vi "File.Read From CSV.vi"(8 "error in":errorcluster, 11 "File":path) -> (0 "error out":errorcluster, 2 "Data":string[][](array[string]), 3 "Header":string[](array[string]))   [LabVIEW 2024, in "EQMF.lvlib" / "File Utils.lvlib"]
uses:
  File Utils.lvlib
  <vilib>/Utility/error.llb/Trim Whitespace One-Sided.vi
panel:
  in  "Has Header Row":bool=TRUE
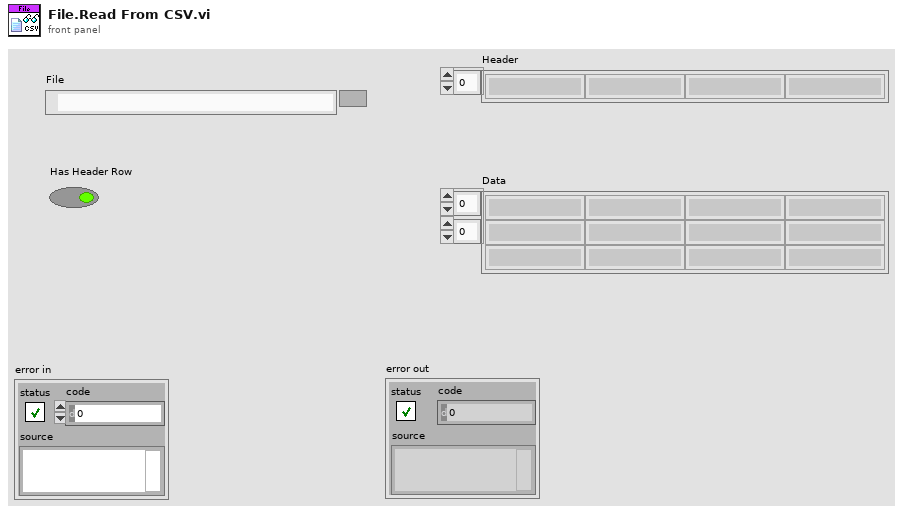
[diagram p1: front panel]
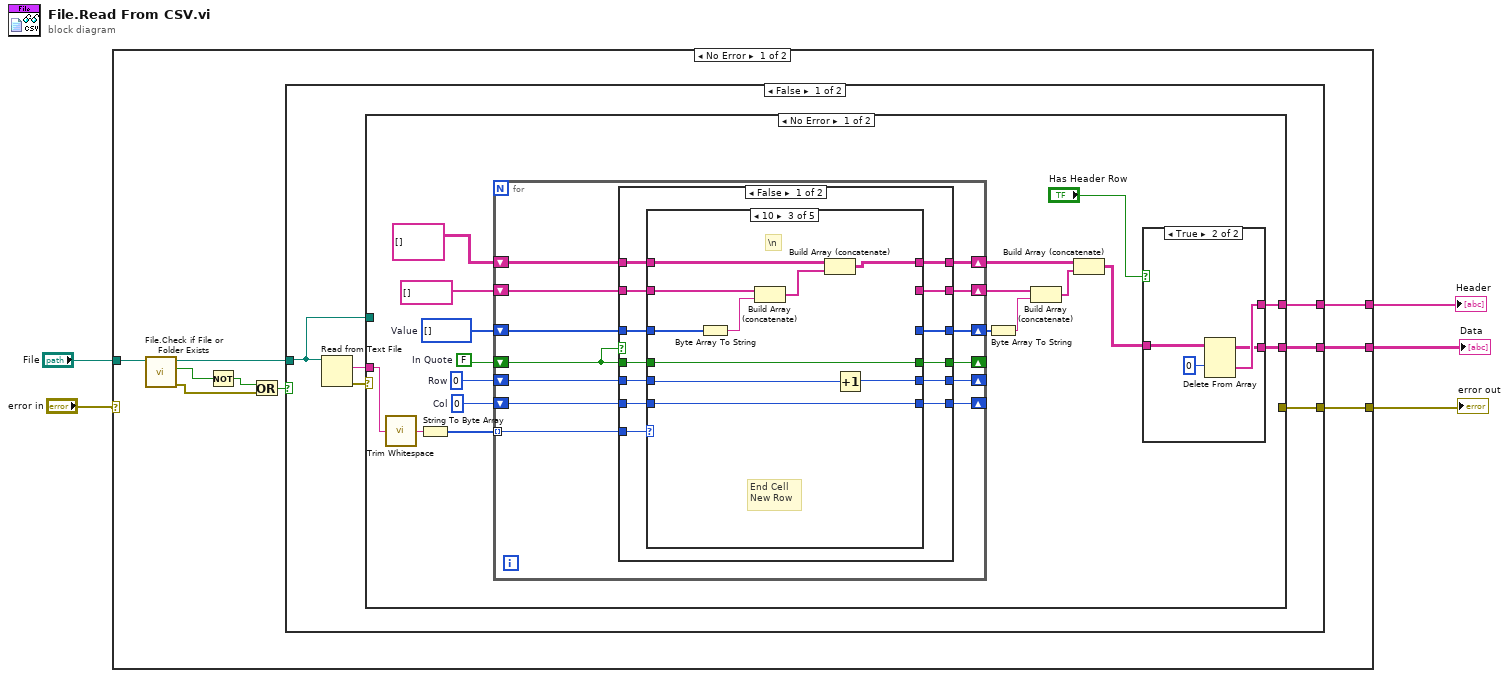
[diagram p0: block diagram]
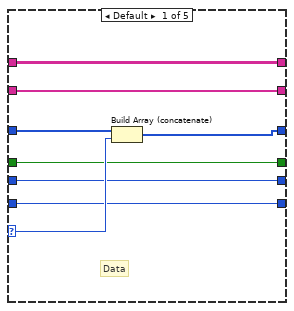
[diagram p2: hidden frame]
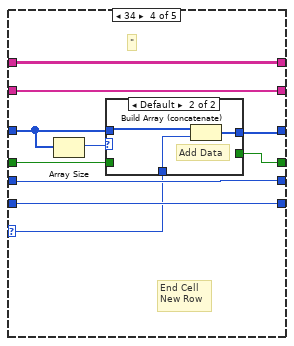
[diagram p4: hidden frame]
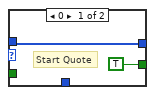
[diagram p5: hidden frame]
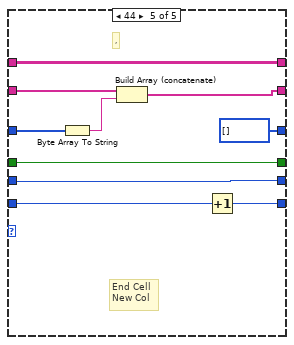
[diagram p6: hidden frame]
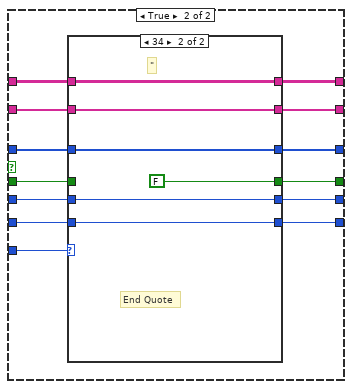
[diagram p7: hidden frame]
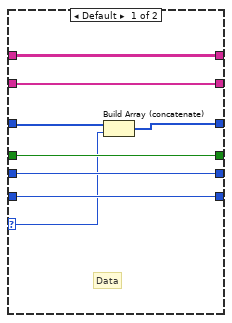
[diagram p8: hidden frame]
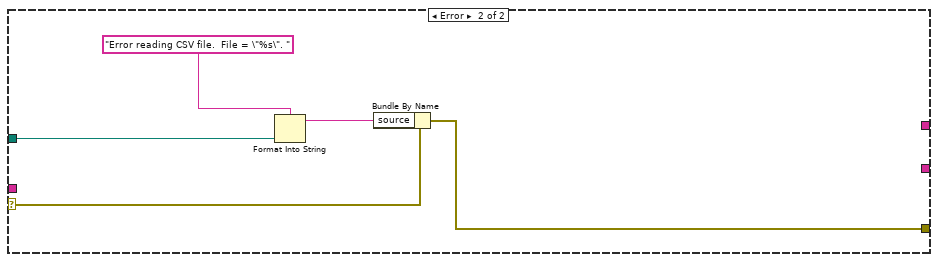
[diagram p10: hidden frame]
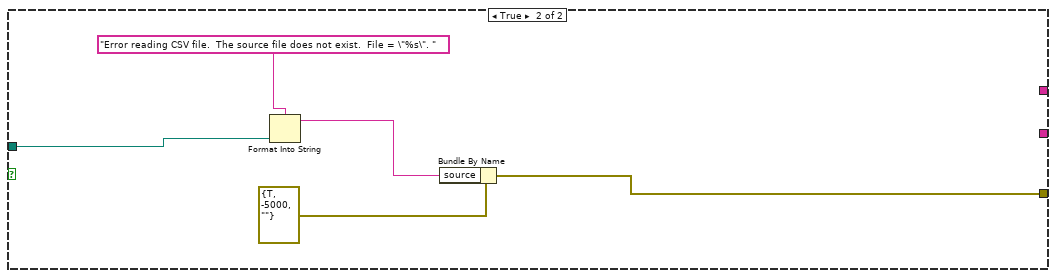
[diagram p11: hidden frame]
diagram:
  n1 = case shown="No Error" "error in" {
    selector: "error in" -> [_ w156]
    tunnel: "File" -> [w14 _]
    tunnel: [w8 w156] -> w3
    tunnel: [w7 _] -> w2
    tunnel: [w6 _] -> w1
    frame No Error {
      n2 = call "File.Check if File or Folder Exists.vi"("Path"=w14) -> ("error out"=w13:errorcluster, "Exists"=w10:bool, "Dup Path"=w11:path)  [unwired: 6 in, 2 out]
      n3 = Not(x=w10) -> (.not. x?=w12:bool)
      n4 = Or(x=w12, y=w13) -> (x .or. y?=w9:bool)
      n5 = case shown="False" w9 {
        tunnel: w11 -> [w18 w154]
        tunnel: [w17 w151] -> w8
        tunnel: [w16 _] -> w7
        tunnel: [w15 _] -> w6
        frame False {
          n6 = Read from Text File(file (use dialog)=w18) -> (text=w19:string, error out=w20:errorcluster)  [unwired: 3 in, 2 out]
          n7 = case shown="No Error" w20 {
            selector: w20 -> [_ w147]
            tunnel: w19 -> [w25 _]
            tunnel: w18 -> [_ w149]
            tunnel: [_ w146] -> w17
            tunnel: [w37 _] -> w16
            tunnel: [w36 _] -> w15
            frame No Error {
              w31 = FALSE  # In Quote
              w32 = u8[] []  # Value
              w33 = 0  # Col
              w34 = 0  # Row
              n8 = call <vilib>:"Trim Whitespace.vi"("string"=w25) -> ("trimmed string"=w26:string)  [unwired: 1 in]
              n9 = String To Byte Array(string=w26) -> (unsigned byte array=w27:u8[])
              n10 = for {
                tunnel: w27 -> [w44] mode=indexing
                shift-right: [w46] -> _
                shift-left: w33 -> [w50]
                shift-right: [w47] -> _
                shift-left: w34 -> [w51]
                shift-right: [w48] -> w23
                shift-left: w32 -> [w49]
                shift-right: [w45] -> _
                shift-left: w31 -> [w43]
                shift-right: [w41] -> w29
                shift-left: string[][] [] ("Raw") -> [w42]
                shift-right: [w40] -> w22
                shift-left: string[] [] ("Raw") -> [w39]
                n11 = case shown="False" w43 {
                  tunnel: w51 -> [w61 w124]
                  tunnel: w50 -> [w60 w122]
                  tunnel: w49 -> [w62 w126]
                  tunnel: [w57 w125] -> w48
                  tunnel: [w56 w123] -> w47
                  tunnel: [w53 w121] -> w46
                  tunnel: [w54 w120] -> w45
                  tunnel: w44 -> [w52 w114]
                  tunnel: w43 -> [w55 w119]
                  tunnel: w42 -> [w64 w116]
                  tunnel: [w63 w115] -> w41
                  tunnel: w39 -> [w58 w118]
                  tunnel: [w59 w117] -> w40
                  frame False {
                    n12 = case shown="10" w52 {
                      selector: w52 -> [w68 _ _ w90 _]
                      tunnel: w64 -> [w72 w78 w88 w96 w109]
                      tunnel: [w72 w78 w87 w96 w109] -> w63
                      tunnel: w62 -> [w70 w73 w79 w94 w110]
                      tunnel: w61 -> [w67 w76 w84 w97 w107]
                      tunnel: w60 -> [w66 w75 w83 w98 w105]
                      tunnel: w58 -> [w71 w77 w81 w95 w111]
                      tunnel: [w71 w77 _ w95 w108] -> w59
                      tunnel: [w69 w73 _ w91 u8[] [] ("Value")] -> w57
                      tunnel: [w67 w76 w85 w97 w107] -> w56
                      tunnel: w55 -> [w65 w74 w86 w92 w113]
                      tunnel: [w65 w74 w86 w89 w113] -> w54
                      tunnel: [w66 w75 w83 w98 w106] -> w53
                      frame Default {
                        # "Data"
                        n13 = Build Array (concatenate)(w70, w68) -> (w69:u8[])
                      }
                      frame 0..9, 11..31 {
                        # "Ignore"
                      }
                      frame 10 {
                        # "\\n"
                        # "End Cell\nNew Row"
                        n14 = Byte Array To String(unsigned byte array=w79) -> (string=w82:string)
                        n15 = Build Array (concatenate)(w81, w82) -> (w80:string[])
                        n16 = Build Array (concatenate)(w88, w80) -> (w87:string[][])
                        n17 = Increment(x=w84) -> (x+1=w85:i32)
                      }
                      frame 34 {
                        # "\""
                        # "End Cell\nNew Row"
                        n18 = Array Size(array=w94) -> (size(s)=w93:i32)
                        n19 = case shown="Default" w93 {
                          tunnel: w94 -> [w99 w103]
                          tunnel: w92 -> [_ _]
                          tunnel: [w99 w102] -> w91
                          tunnel: w90 -> [_ w101]
                          tunnel: [TRUE _] -> w89
                          frame 0 {
                            # "Start Quote"
                          }
                          frame Default {
                            # "Add Data"
                            n20 = Build Array (concatenate)(w103, w101) -> (w102:u8[])
                          }
                        }
                      }
                      frame 44 {
                        # ","
                        # "End Cell\nNew Col"
                        n21 = Byte Array To String(unsigned byte array=w110) -> (string=w112:string)
                        n22 = Build Array (concatenate)(w111, w112) -> (w108:string[])
                        n23 = Increment(x=w105) -> (x+1=w106:i32)
                      }
                    }
                  }
                  frame True {
                    n24 = case shown="34" w114 {
                      selector: w114 -> [w127 _]
                      tunnel: w126 -> [w132 w140]
                      tunnel: [w131 w140] -> w125
                      tunnel: w124 -> [w133 w139]
                      tunnel: [w133 w139] -> w123
                      tunnel: w122 -> [w134 w138]
                      tunnel: [w134 w138] -> w121
                      tunnel: [w130 FALSE] -> w120
                      tunnel: w119 -> [w130 _]
                      tunnel: w118 -> [w128 w136]
                      tunnel: [w128 w136] -> w117
                      tunnel: w116 -> [w129 w135]
                      tunnel: [w129 w135] -> w115
                      frame Default {
                        # "Data"
                        n25 = Build Array (concatenate)(w132, w127) -> (w131:u8[])
                      }
                      frame 34 {
                        # "\""
                        # "End Quote"
                      }
                    }
                  }
                }
              }
              n26 = Byte Array To String(unsigned byte array=w23) -> (string=w24:string)
              n27 = Build Array (concatenate)(w22, w24) -> (w21:string[])
              n28 = Build Array (concatenate)(w29, w21) -> (w28:string[][])
              n29 = case shown="True" "Has Header Row" {
                tunnel: w28 -> [w141 w145]
                tunnel: [_ w143] -> w37
                tunnel: [w141 w142] -> w36
                frame False {
                }
                frame True {
                  n30 = Delete From Array(array=w145, index (row)=0 ("length")) -> (deleted portion=w143:string[], array with subset deleted=w142:string[][])  [unwired: 2 in]
                }
              }
            }
            frame Error {
              n31 = Format Into String(format string="Error reading CSV file.  File = \"%s\". ", w149) -> (resulting string=w148:string)  [unwired: 2 in, 1 out]
              n32 = Bundle By Name(cluster=w147, "source"=w148) -> (w146:errorcluster)
            }
          }
        }
        frame True {
          n33 = Format Into String(format string="Error reading CSV file.  The source file does not exist.  File = \"%s\". ", w154) -> (resulting string=w152:string)  [unwired: 2 in, 1 out]
          n34 = Bundle By Name(cluster=errorcluster {"status"=TRUE, "code"=-5000, "source"=""} ("error constant"), "source"=w152) -> (w151:errorcluster)
        }
      }
    }
    frame Error {
    }
  }
  "error out" <- w3
  "Header" <- w2
  "Data" <- w1
